vi "XNode Demo.vi"   [LabVIEW 2018]
uses:
  Array Dimension Array/Array Dimension Array.xnode
  ArrayDimension/ArrayDimension.xnode
  Unindex and unbundle/Unindex and Unbundle.xnode
  Filter Array/FilterArray.xnode
  Foreign Key Sort/Foreign Key Sort.xnode
  Minimum Array Size/Minimum Array Size.xnode
  Array Size and Index/Array Size and Index.xnode
  Shuffle Array/Shuffle Array.xnode
  <vilib>/Analysis/1siggen.llb/Ramp Pattern.vi
  <vilib>/Analysis/NI_AALBase.lvlib
  <vilib>/Analysis/1siggen.llb/Ramp Pattern by Samples.vi
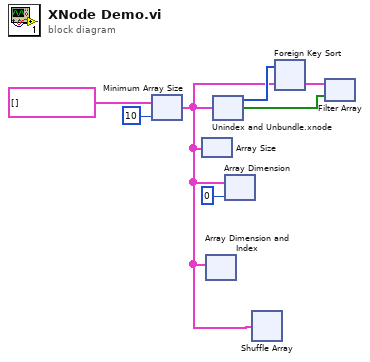
[diagram p0: block diagram]
diagram:
  n1 = xnode "Minimum Array Size"("Array In"=cluster{i32, bool, string}[] [], "Size"=10) -> ("Array Out"=w1:cluster{i32, bool, string}[])
  n2 = xnode "Array Size"("Array"=w1) -> ()  [unwired: 1 out]
  n3 = xnode "Array Dimension and Index"("Array In"=w1) -> ()  [unwired: 1 out]
  n4 = xnode "Unindex and Unbundle.xnode"("array of clusters (xi,yi, ..."=w1) -> ("Element 0"=w5:i32[], "Element 1"=w3:bool[])  [unwired: 1 out]
  n5 = xnode "Array Dimension"("Array"=w1, "Dimension"=0) -> ()  [unwired: 1 out]
  n6 = xnode "Shuffle Array"("Array In"=w1) -> ()  [unwired: 1 out]
  n7 = xnode "Foreign Key Sort"("Keys"=w5, "Array"=w1) -> ("Sorted Array"=w4:cluster{i32, bool, string}[])  [unwired: 1 out]
  n8 = xnode "Filter Array"("Array"=w4, "Filter?"=w3) -> ()  [unwired: 2 out]
